vi "FTW-DevUtil-FindClones.vi"(0 "Application in":refnum<vi>, 1 "Search Clones Up To":i32=100, 7 "VIs in":string[](array[string])) -> (8 "VIs (including clones) out":string[](array[string]))   [LabVIEW 2013]
doc: "Given a list of VIs in memory, and belonging to a particular Application Instance; this VI returns the input list, plus up to N instances of all statically-referenced clones currently in memory. The clones are enumerated.\n\nLabVIEW Task Manager v1.7.0.28\nRavi Beniwal (packaged by TimVargo) - LAVA\nCopyright (c) 2011-2014, Ravi Beniwal"
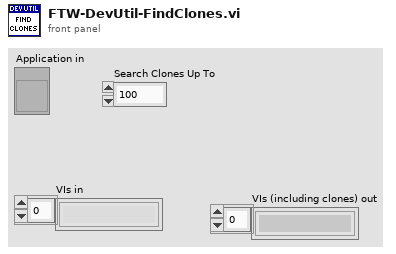
[diagram p1: front panel]
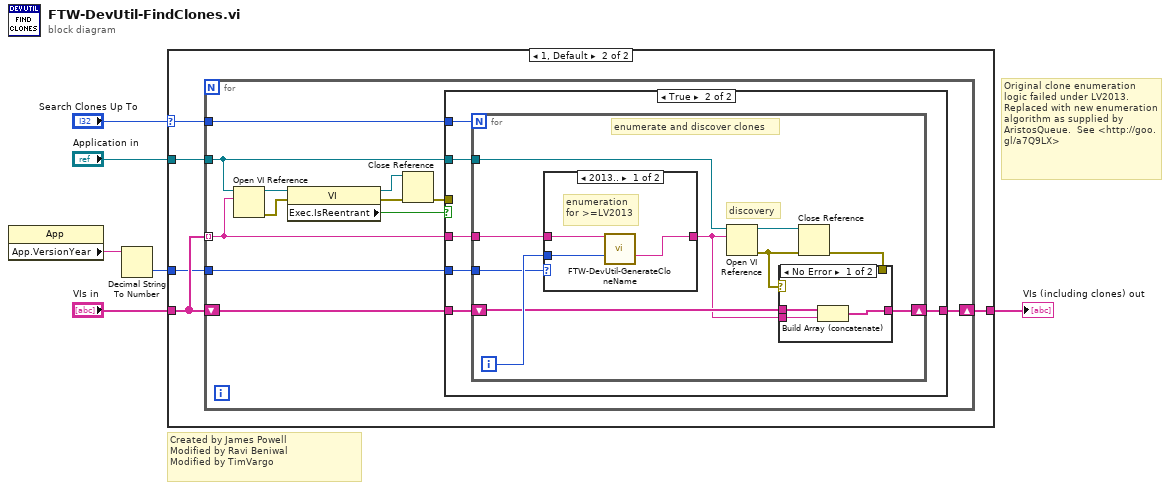
[diagram p0: block diagram]
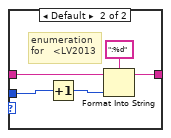
[diagram p4: hidden frame]
diagram:
  # "Original clone enumeration logic failed under LV2013.  Replaced with new enumeration algorithm as supplied by AristosQueue.  See <http://goo.gl/a7Q9LX>"
  # "Created by James Powell\nModified by Ravi Beniwal\nModified by TimVargo"
  n1 = property class="App"() -> ("App.VersionYear"=w2:string)  [unwired: 2 in, 2 out]
  n2 = Decimal String To Number(string=w2) -> (number=w1:i32)  [unwired: 2 in, 1 out]
  n3 = case shown="1, Default" "Search Clones Up To" {
    selector: "Search Clones Up To" -> [_ w9]
    tunnel: [w7 w12] -> w6
    tunnel: "Application in" -> [_ w11]
    tunnel: "VIs in" -> [w7 w10]
    tunnel: w1 -> [_ w8]
    frame 0 {
    }
    frame 1, Default {
      n4 = for {
        tunnel: w10 -> [w18] mode=indexing
        tunnel: w11 -> [w19]
        shift-right: [w17] -> w12
        shift-left: w10 -> [w15]
        tunnel: w9 -> [w16]
        tunnel: w8 -> [w13]
        n5 = Open VI Reference(application reference (local)=w19, vi path=w18) -> (vi reference=w23:refnum<vi>, error out=w24:errorcluster)  [unwired: 4 in]
        n6 = property class="VI"(reference=w23, error in=w24) -> (reference out=w22:refnum<vi>, error out=w21:errorcluster, "Exec.IsReentrant"=w20:bool)
        n7 = Close Reference(reference=w22, error in (no error)=w21) -> (error out=w14:errorcluster)
        n8 = case shown="True" w20 {
          tunnel: w18 -> [_ w31]
          tunnel: w19 -> [_ w30]
          tunnel: w15 -> [w25 w29]
          tunnel: [w25 w28] -> w17
          tunnel: w16 -> [_ w27]
          tunnel: w14 -> [_ _]
          tunnel: w13 -> [_ w26]
          frame False {
          }
          frame True {
            n9 = for {
              N: w27 -> [_]
              tunnel: w31 -> [w41]
              tunnel: w30 -> [w37]
              shift-right: [w39] -> w28
              shift-left: w29 -> [w38]
              tunnel: w26 -> [w32]
              i -> [w40]
              # "discovery"
              # "enumerate and discover clones"
              n10 = case shown="2013.." w32 {
                tunnel: w41 -> [w44 w49]
                tunnel: w40 -> [w43 w48]
                tunnel: [w42 w47] -> w34
                frame 2013.. {
                  # "enumeration\nfor >=LV2013"
                  n11 = call "FTW-DevUtil-GenerateCloneName.vi"("Fully qualified VI name"=w44, "Clone number (1)"=w43) -> ("Fully qualified clone name"=w42:string)  [unwired: 11 in, 2 out]
                }
                frame Default {
                  # "enumeration\nfor   <LV2013"
                  n12 = Increment(x=w48) -> (x+1=w45:i32)
                  n13 = Format Into String(format string=":%d", initial string=w49, w45) -> (resulting string=w47:string)  [unwired: 1 in, 1 out]
                }
              }
              n14 = Open VI Reference(application reference (local)=w37, vi path=w34) -> (vi reference=w35:refnum<vi>, error out=w36:errorcluster)  [unwired: 4 in]
              n15 = Close Reference(reference=w35, error in (no error)=w36) -> (error out=w33:errorcluster)
              n16 = case shown="No Error" w36 {
                tunnel: [w52 w53] -> w39
                tunnel: w38 -> [w51 w53]
                tunnel: w34 -> [w50 _]
                tunnel: w33 -> [_ _]
                frame No Error {
                  n17 = Build Array (concatenate)(w51, w50) -> (w52:string[])
                }
                frame Error {
                }
              }
            }
          }
        }
      }
    }
  }
  "VIs (including clones) out" <- w6
